vi "capt_scaling.vi"(7 "Index":i32=250, 8 "error in":errorcluster, 10 "Gain":sgl format="%.6e", 11 "Offset":sgl format="%.6e") -> (0 "error out":errorcluster)   [LabVIEW 2012]
uses:
  GlobalVariables/PT01Parameters.vi
  GlobalVariables/PT02Parameters.vi
  GlobalVariables/PT03Parameters.vi
panel:
  in  "Address":u8=250 format="%x"
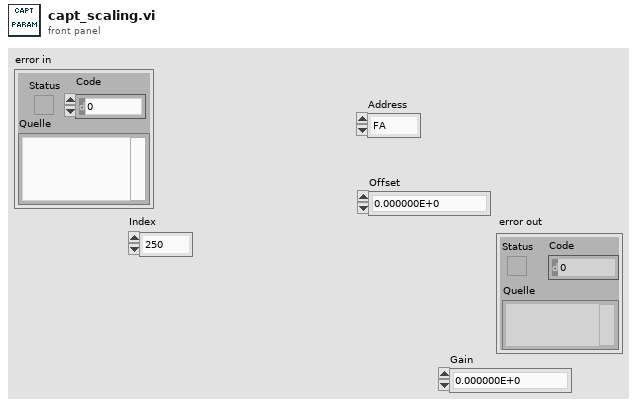
[diagram p1: front panel]
types:
  T1 = cluster{"baudrate":u32, "databits":u16, "paritybit":u16, "stopbits":u16, "flux control":u16, "Port":string, "Register Address":u16, "Serial Parameters":cluster{"Mode":enum16{"RTU", "ASCII"}, "Slave Address":u8}, "Timeout":u32, "PressureLimit":dbl}
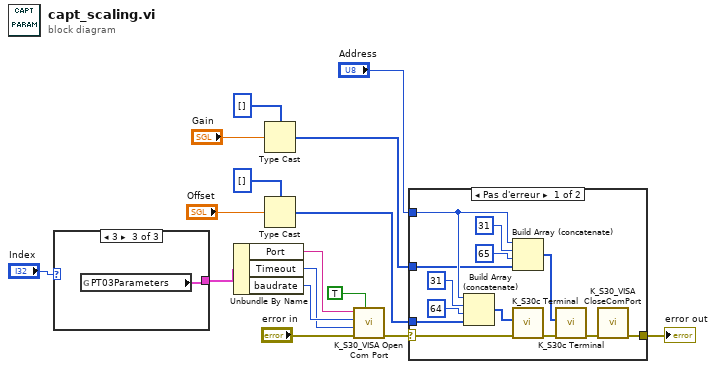
[diagram p0: block diagram]
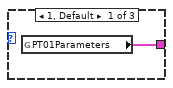
[diagram p2: hidden frame]
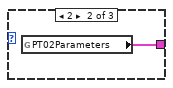
[diagram p3: hidden frame]
diagram:
  n1 = case shown="3" "Index" {
    tunnel: [w17 w18 w19] -> w1
    frame 1, Default {
      n2 = global read "PT01Parameters.vi" "PT01Parameters"() -> (w17:T1)
    }
    frame 2 {
      n3 = global read "PT02Parameters.vi" "PT02Parameters"() -> (w18:T1)
    }
    frame 3 {
      n4 = global read "PT03Parameters.vi" "PT03Parameters"() -> (w19:T1)
    }
  }
  n5 = Unbundle By Name(w1) -> ("Port"=w15:string, "Timeout"=w12:u32, "baudrate"=w14:u32)
  n6 = Type Cast(type=u8[] [] ("response"), x="Gain") -> (*(type *) &x=w3:u8[])
  n7 = Type Cast(type=u8[] [] ("response"), x="Offset") -> (*(type *) &x=w7:u8[])
  n8 = call "K_S30_VISA Open Com Port.vi"("RS-converter:\necho"=TRUE ("RS-converter: echo"), "error in (no error)"="error in", "timeout"=w12, "Baudrate"=w14, "VISA resource name"=w15) -> ("error out"=w6:errorcluster)  [unwired: 3 in, 1 out]
  n9 = case shown="Pas d'erreur" w6 {
    selector: w6 -> [w30 w33]
    tunnel: "Address" -> [w25 _]
    tunnel: [w21 w33] -> w10
    tunnel: w7 -> [w29 _]
    tunnel: w3 -> [w22 _]
    frame No Error {
      n10 = Build Array (concatenate)(w25, u8 31 ("Element"), u8 64 ("Register"), w29) -> (w31:u8[])
      n11 = Build Array (concatenate)(w25, u8 31 ("Element"), u8 65 ("Register"), w22) -> (w26:u8[])
      n12 = call "K_S30c Terminal.vi"("error in"=w30, "request"=w31) -> ("error out"=w28:errorcluster)  [unwired: 4 in, 1 out]
      n13 = call "K_S30c Terminal.vi"("error in"=w28, "request"=w26) -> ("error out"=w20:errorcluster)  [unwired: 4 in, 1 out]
      n14 = call "K_S30_VISA CloseComPort.vi"("error in (not connected)"=w20) -> ("Fehlerausgang"=w21:errorcluster)  [unwired: 6 in]
    }
    frame Error {
    }
  }
  "error out" <- w10
